vi "Calc Frequency-RMS-Pk-Pk.vi"(0 "Signal Data In":sgl[](array[numeric]), 1 "Sample Rate":dbl) -> (15 "RMS":dbl[](array[numeric]), 16 "Pk-Pk":dbl[](array[numeric]), 17 "Frequency":dbl[](array[numeric]), 18 "Peak":dbl[](array[numeric]), 19 "Valley":dbl[](array[numeric]))   [LabVIEW 2013]
uses:
  <vilib>/Analysis/baseanly.llb/Mean (DBL).vi
  <vilib>/ptbypt/NI_PtbyPt.lvlib
  <vilib>/Analysis/NI_AALBase.lvlib
panel:
  out "Waveform Chart 2":dbl[](graph)
  out "Waveform Chart":dbl[][](graph)
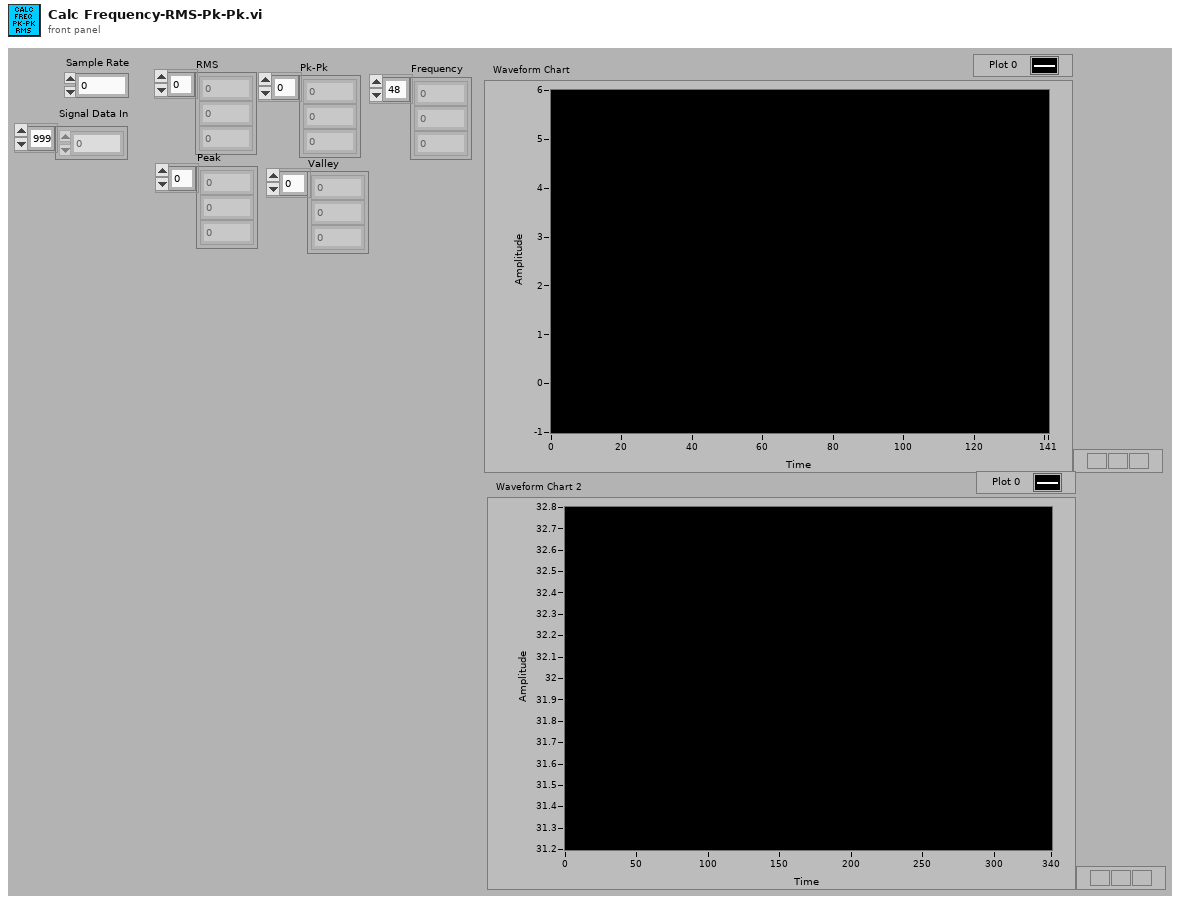
[diagram p1: front panel]
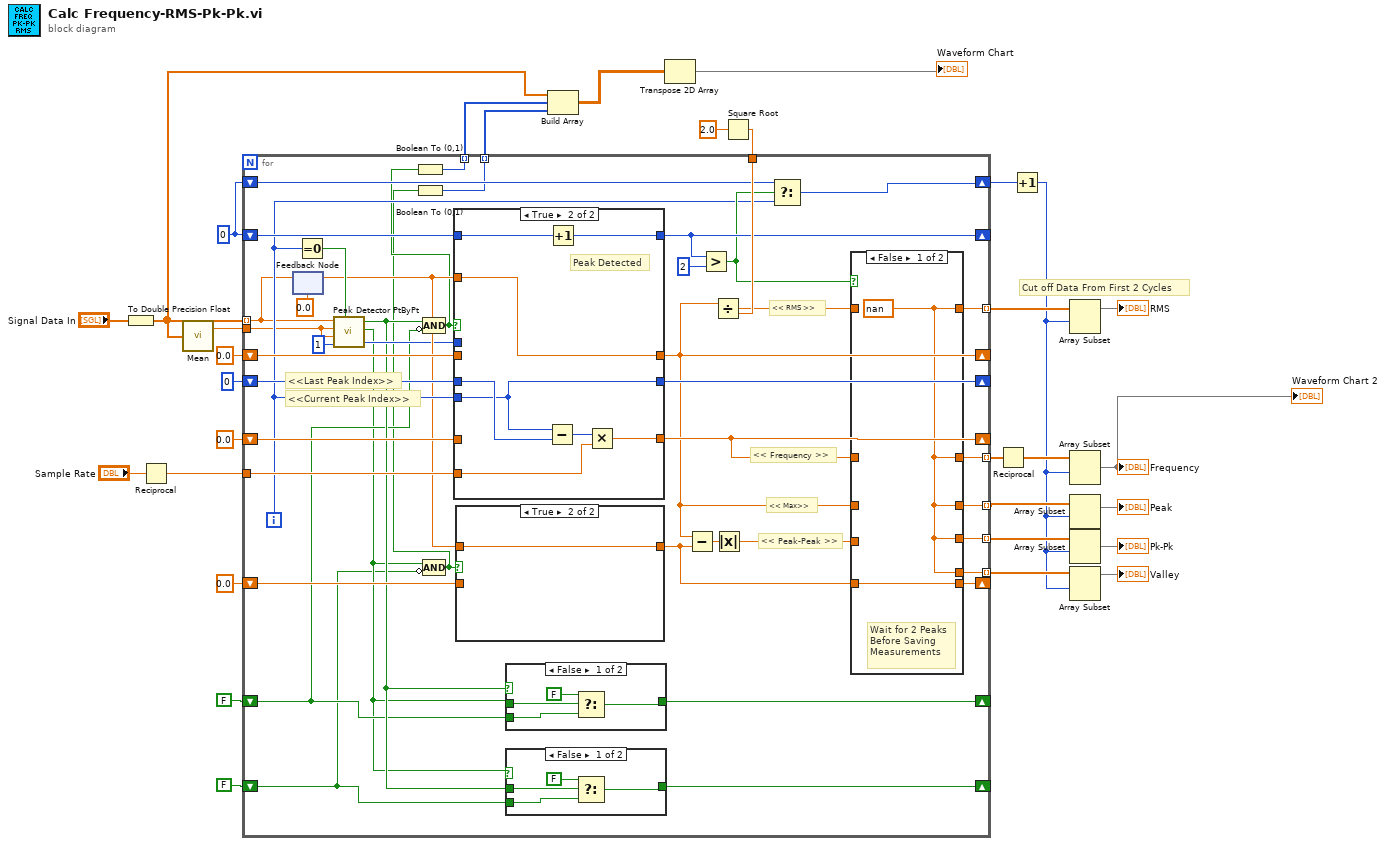
[diagram p0: block diagram]
diagram:
  w22 = 0
  # "Cut off Data From First 2 Cycles"
  n1 = To Double Precision Float(number="Signal Data In") -> (double precision float=w8:dbl[])
  n2 = Reciprocal(x="Sample Rate") -> (1/x=w24:dbl)
  n3 = call-poly <vilib>:"Mean.vi"("X"=w8) -> ("mean"=w19:dbl)  [unwired: 1 out]
  n4 = Square Root(x=2.0) -> (sqrt(x)=w27:dbl)
  n5 = for {
    tunnel: w8 -> [w43] mode=indexing
    shift-right: [w50] -> _
    shift-left: 0.0 -> [w73]
    shift-right: [w61] -> _
    shift-left: 0 -> [w72]
    tunnel: w24 -> [w71]
    shift-right: [w66] -> _
    shift-left: 0.0 -> [w70]
    tunnel: [w65] -> w26 mode=indexing
    tunnel: w27 -> [w69]
    tunnel: [w67] -> w25 mode=indexing
    shift-right: [w63] -> _
    shift-left: w22 -> [w64]
    shift-right: [w57] -> w20
    shift-left: w22 -> [w58]
    tunnel: w19 -> [w42]
    shift-right: [w47] -> _
    shift-left: 0.0 -> [w54]
    tunnel: [w52] -> w15 mode=indexing
    tunnel: [w49] -> w14 mode=indexing
    tunnel: [w46] -> w12 mode=indexing
    tunnel: [w45] -> w9 mode=indexing
    tunnel: [w44] -> w5 mode=indexing
    shift-right: [w40] -> _
    shift-left: FALSE -> [w36]
    shift-right: [w39] -> _
    shift-left: FALSE -> [w34]
    i -> [w59]
    # "<< Max>>"
    # "<< Peak-Peak >>"
    # "<<Last Peak Index>>"
    # "<<Current Peak Index>>"
    # "<< RMS >>"
    # "<< Frequency >>"
    n6 = feedback-in #1(w43) -> ()
    n7 = feedback #1(0.0) -> (w55:dbl)
    n8 = Equal To 0?(x=w59) -> (x = 0?=w74:bool)
    n9 = call <vilib>:"Peak Detector PtByPt.vi"("x"=w43, "threshold peak"=w42, "threshold valley"=w42, "width"=1, "initialize"=w74) -> ("peak"=w38:bool, "valley"=w35:bool, "error"=w41:i32)
    n10 = Compound Arithmetic op=AND(w38, invert w36) -> (w37:bool)
    n11 = Boolean To (0,1)(Boolean=w37) -> (0, 1=w45:i16)
    n12 = Compound Arithmetic op=AND(w35, invert w34) -> (w33:bool)
    n13 = Boolean To (0,1)(Boolean=w33) -> (0, 1=w44:i16)
    n14 = case shown="True" w37 {
      tunnel: w55 -> [_ w105]
      tunnel: [w97 w105] -> w50
      tunnel: w73 -> [w97 _]
      tunnel: [w96 w98] -> w61
      tunnel: w59 -> [_ w98]
      tunnel: w72 -> [w96 w101]
      tunnel: w71 -> [_ w103]
      tunnel: [w95 w102] -> w66
      tunnel: w70 -> [w95 _]
      tunnel: [w94 w99] -> w63
      tunnel: w64 -> [w94 w100]
      tunnel: w41 -> [_ _]
      frame False {
        # "No Peak"
      }
      frame True {
        # "Peak Detected"
        n15 = Subtract(x=w98, y=w101) -> (x-y=w104:i32)
        n16 = Increment(x=w100) -> (x+1=w99:i32)
        n17 = Multiply(x=w104, y=w103) -> (x*y=w102:dbl)
      }
    }
    n18 = case shown="True" w33 {
      tunnel: w55 -> [_ w86]
      tunnel: w54 -> [w85 _]
      tunnel: [w85 w86] -> w48
      frame False {
      }
      frame True {
      }
    }
    n19 = case shown="False" w38 {
      selector: w38 -> [_ w84]
      tunnel: [w80 w84] -> w40
      tunnel: w35 -> [w83 _]
      tunnel: w36 -> [w81 _]
      frame False {
        n20 = Select(t=FALSE, s=w83, f=w81) -> (s? t:f=w80:bool)
      }
      frame True {
      }
    }
    n21 = case shown="False" w35 {
      selector: w35 -> [_ w79]
      tunnel: [w75 w79] -> w39
      tunnel: w38 -> [w78 _]
      tunnel: w34 -> [w76 _]
      frame False {
        n22 = Select(t=FALSE, s=w78, f=w76) -> (s? t:f=w75:bool)
      }
      frame True {
      }
    }
    n23 = Subtract(x=w50, y=w48) -> (x-y=w53:dbl)
    n24 = Greater?(x=w63, y=2) -> (0:w60:bool)
    n25 = Divide(x=w50, y=w69) -> (x/y=w68:dbl)
    n26 = Absolute Value(x=w53) -> (abs(x)=w51:dbl)
    n27 = Select(t=w58, s=w60, f=w59) -> (s? t:f=w57:i32)
    n28 = case shown="False" w60 {
      tunnel: w68 -> [_ w93]
      tunnel: [w87 w93] -> w67
      tunnel: w66 -> [_ w92]
      tunnel: [w87 w92] -> w65
      tunnel: [w87 w91] -> w52
      tunnel: w51 -> [_ w91]
      tunnel: w50 -> [_ w90]
      tunnel: [w87 w90] -> w49
      tunnel: [w88 w89] -> w47
      tunnel: w48 -> [w88 w89]
      tunnel: [w87 w89] -> w46
      frame False {
        w87 = nan
        # "Wait for 2 Peaks\nBefore Saving\nMeasurements"
        # "Wait for 2 Peaks\nBefore Saving\nMeasurements"
      }
      frame True {
        # "More then 2\nCycles Detected"
      }
    }
  }
  n29 = Build Array(w8, w9, w5) -> (w7:dbl[][])
  n30 = Transpose 2D Array(2D array=w7) -> (transposed array=→"Waveform Chart":dbl[][])
  n31 = Reciprocal(x=w26) -> (1/x=w18:dbl[])
  n32 = Increment(x=w20) -> (x+1=w11:i32)
  n33 = Array Subset(array=w25, index=w11) -> (→"RMS":dbl[])  [unwired: 1 in]
  n34 = Array Subset(array=w18, index=w11) -> (→"Frequency" →"Waveform Chart 2":dbl[])  [unwired: 1 in]
  n35 = Array Subset(array=w14, index=w11) -> (→"Peak":dbl[])  [unwired: 1 in]
  n36 = Array Subset(array=w15, index=w11) -> (→"Pk-Pk":dbl[])  [unwired: 1 in]
  n37 = Array Subset(array=w12, index=w11) -> (→"Valley":dbl[])  [unwired: 1 in]
